vi "Alarme_Geral.vi"() -> ()   [LabVIEW 2019]
panel:
  out "ALARME":bool
  in  "CODIGO":string
  out "DESCRI敲O DO ERRO:":string
  out "STR_ALARME:":string
  in  "[ESC]":bool
  # "ALARME"
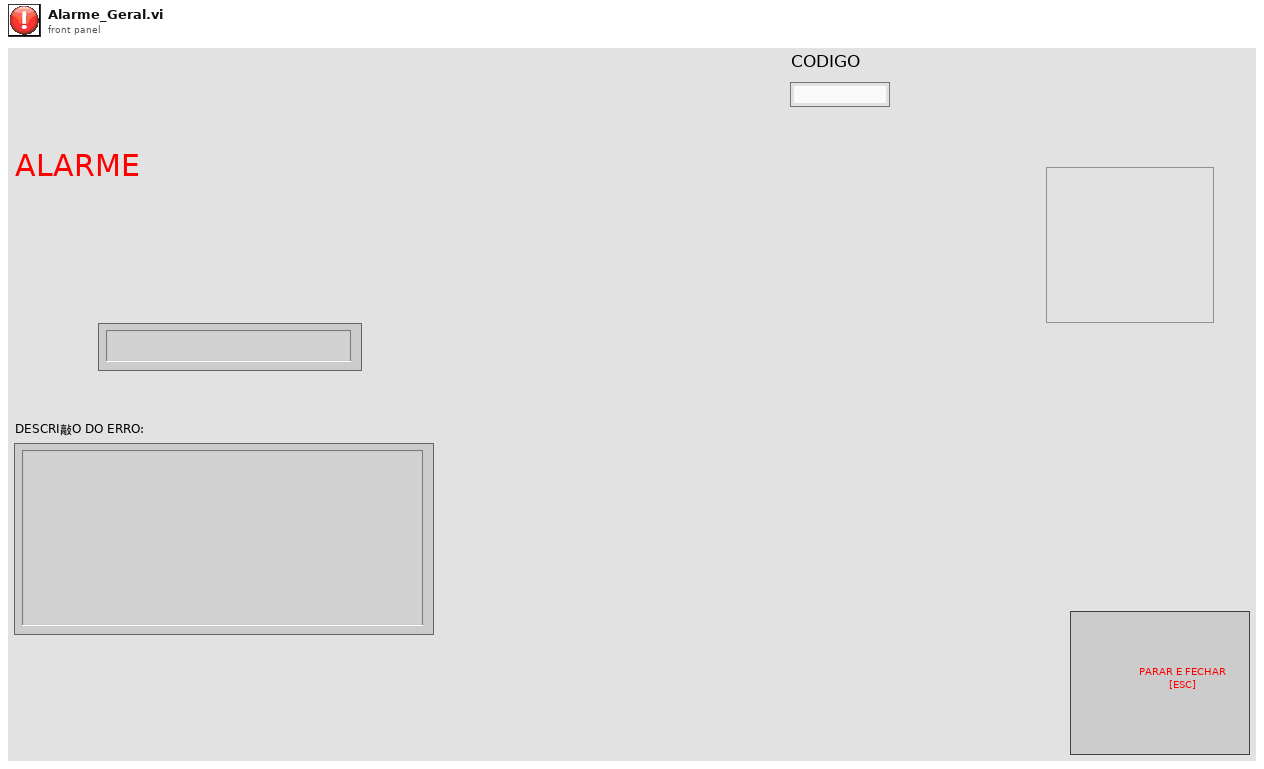
[diagram p1: front panel]
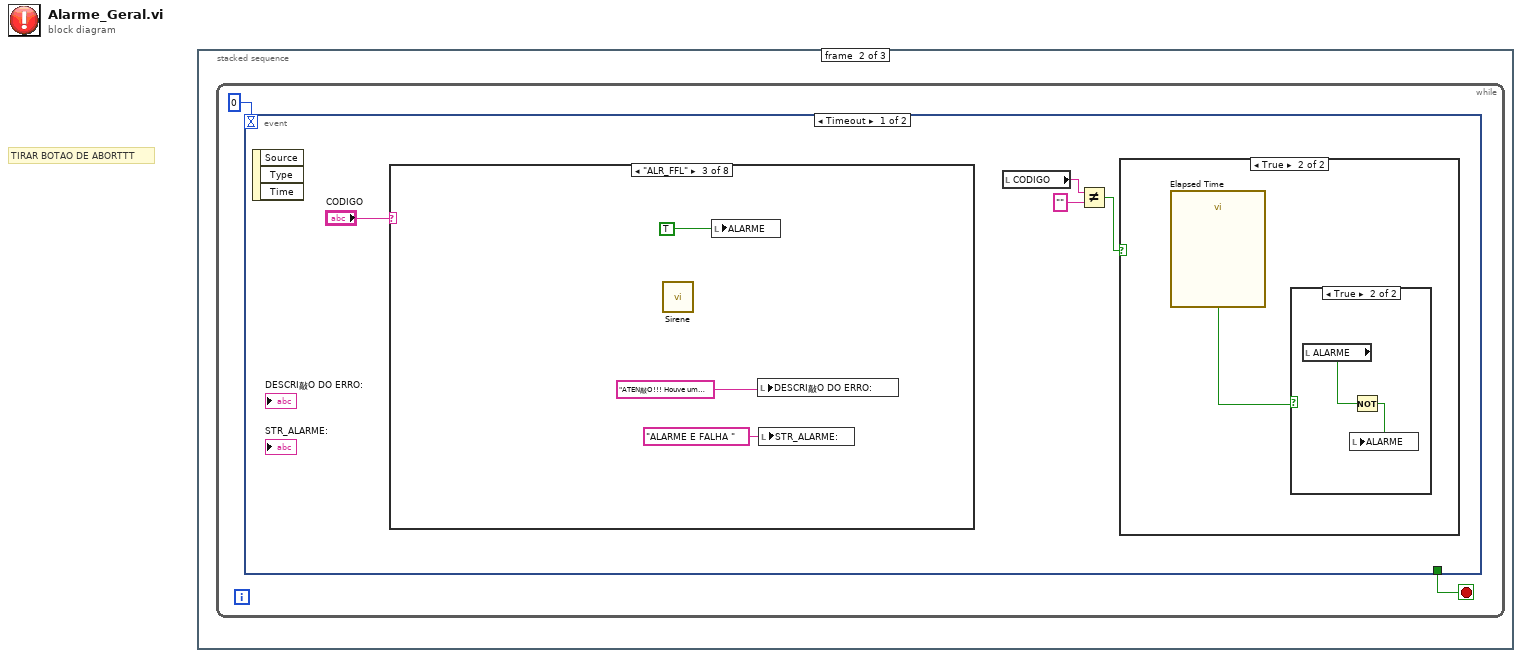
[diagram p0: block diagram]
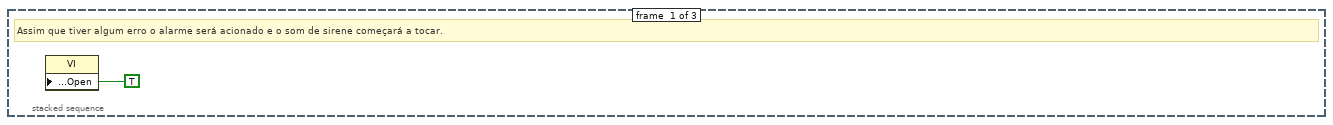
[diagram p2: hidden frame]
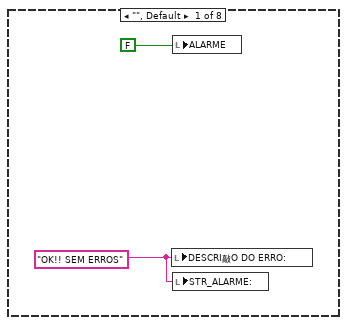
[diagram p5: hidden frame]
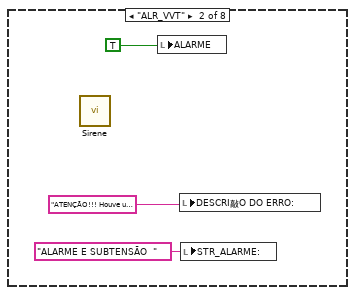
[diagram p6: hidden frame]
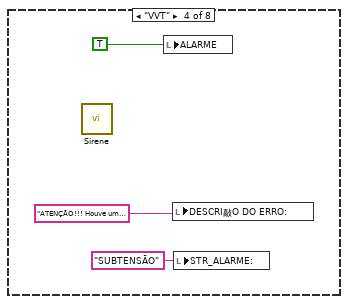
[diagram p7: hidden frame]
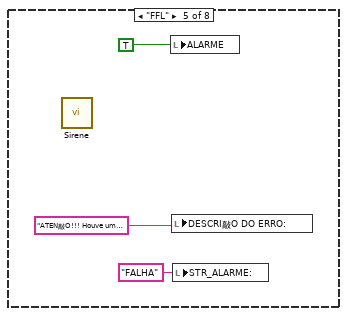
[diagram p8: hidden frame]
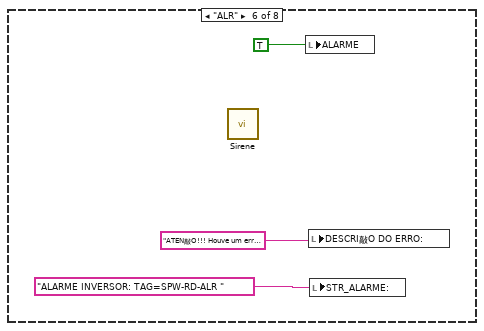
[diagram p9: hidden frame]
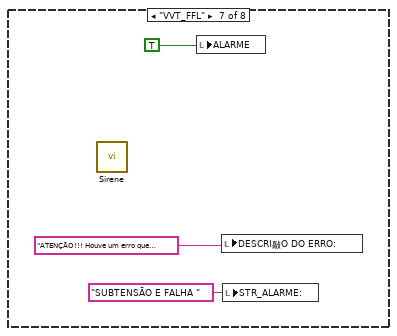
[diagram p10: hidden frame]
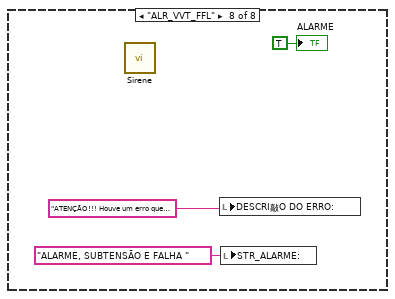
[diagram p11: hidden frame]
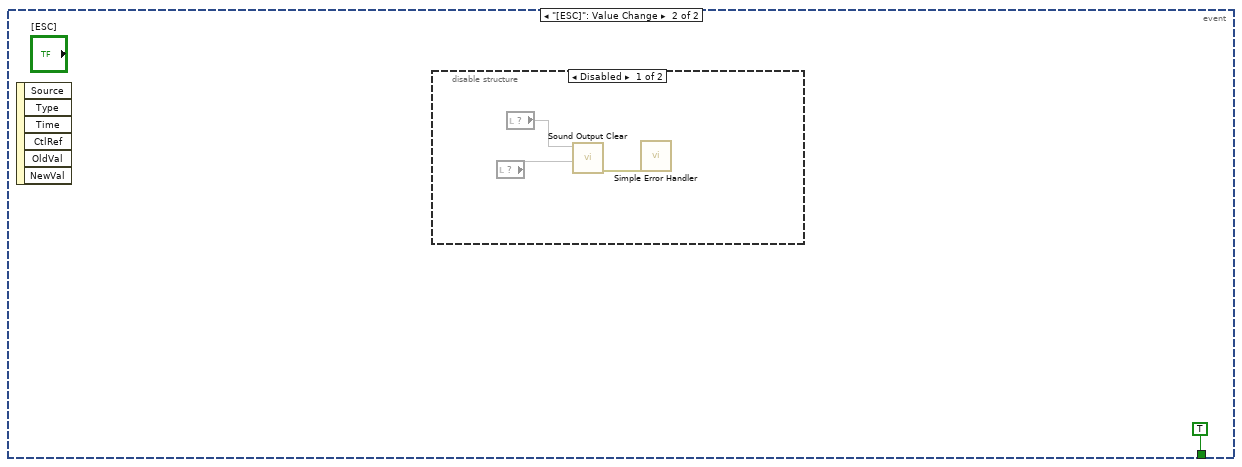
[diagram p12: hidden frame]
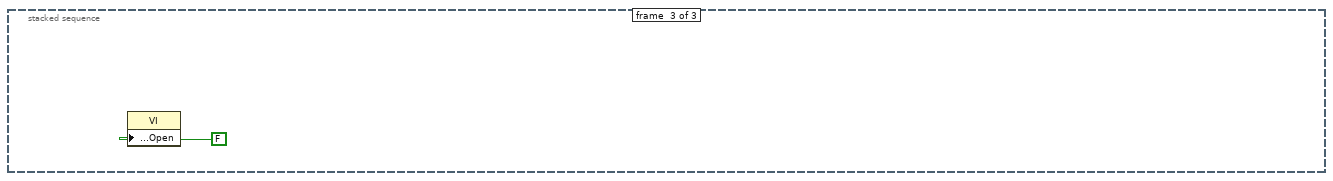
[diagram p14: hidden frame]
diagram:
  # "TIRAR BOTAO DE ABORTTT"
  n1 = stacked-sequence {
    frame #0 {
      # "Assim que tiver algum erro o alarme será acionado e o som de sirene começará a tocar."
      n2 = property class="VI"("Front Panel.Open"=TRUE ("Front Panel Window:Open")) -> ()  [unwired: 2 in, 2 out]
    }
    frame #1 {
      n3 = while {
        stop <- w2 stop-if-true
        n4 = event shown="[0] Timeout" {
          selector: _ -> [_ _]
          dyn-events: _ -> [_ _]
          timeout: 0 -> [_ _]
          tunnel: [_ TRUE] -> w2
          event Timeout {
            n5 = event-data() -> ()  [unwired: 1 in, 3 out]
            n6 = case shown="\"ALR_FFL\"" "CODIGO" {
              frame "", Default {
                w11 = "OK!! SEM ERROS" ("DESCRI敲O DO ERRO:")
                n7 = local write "DESCRI敲O DO ERRO:"(w11) -> ()
                n8 = local write "ALARME"(FALSE ("Alarme_button")) -> ()
                n9 = local write "STR_ALARME:"(w11) -> ()
              }
              frame "ALR_VVT" {
                n10 = call "Sirene.vi"() -> ()  [unwired: 12 in]
                n11 = local write "ALARME"(TRUE ("Alarme_button")) -> ()
                n12 = local write "DESCRI敲O DO ERRO:"("ATENÇÃO!!! Houve um erro que disparou o alarme e o alerta de subtensão. Cheque os parametros e as possiveis causas. " ("DESCRI敲O DO ERRO:")) -> ()
                n13 = local write "STR_ALARME:"("ALARME E SUBTENSÃO  " ("STR_ALARME:")) -> ()
              }
              frame "ALR_FFL" {
                n14 = call "Sirene.vi"() -> ()  [unwired: 12 in]
                n15 = local write "ALARME"(TRUE ("Alarme_button")) -> ()
                n16 = local write "DESCRI敲O DO ERRO:"("ATEN敲O!!! Houve um erro que disparou o alarme e a falha. Cheque os parametros e as possiveis causas. " ("DESCRI敲O DO ERRO:")) -> ()
                n17 = local write "STR_ALARME:"("ALARME E FALHA " ("STR_ALARME:")) -> ()
              }
              frame "VVT" {
                n18 = call "Sirene.vi"() -> ()  [unwired: 12 in]
                n19 = local write "ALARME"(TRUE ("Subtensao_button")) -> ()
                n20 = local write "DESCRI敲O DO ERRO:"("ATENÇÃO!!! Houve um erro que disparou o alerta de subtensão. Cheque os parametros e as possiveis causas. " ("DESCRI敲O DO ERRO:")) -> ()
                n21 = local write "STR_ALARME:"("SUBTENSÃO" ("STR_ALARME:")) -> ()
              }
              frame "FFL" {
                n22 = call "Sirene.vi"() -> ()  [unwired: 12 in]
                n23 = local write "ALARME"(TRUE ("Alarme_button")) -> ()
                n24 = local write "DESCRI敲O DO ERRO:"("ATEN敲O!!! Houve um erro que disparou a falha. Cheque os parametros e as possiveis causas. " ("DESCRI敲O DO ERRO:")) -> ()
                n25 = local write "STR_ALARME:"("FALHA" ("STR_ALARME:")) -> ()
              }
              frame "ALR" {
                n26 = call "Sirene.vi"() -> ()  [unwired: 12 in]
                n27 = local write "ALARME"(TRUE ("Alarme_button")) -> ()
                n28 = local write "DESCRI敲O DO ERRO:"("ATEN敲O!!! Houve um erro que disparou o alerta. Cheque os parametros e as possiveis causas. " ("DESCRI敲O DO ERRO:")) -> ()
                n29 = local write "STR_ALARME:"("ALARME INVERSOR: TAG=SPW-RD-ALR " ("STR_ALARME:")) -> ()
              }
              frame "VVT_FFL" {
                n30 = call "Sirene.vi"() -> ()  [unwired: 12 in]
                n31 = local write "ALARME"(TRUE ("Alarme_button")) -> ()
                n32 = local write "DESCRI敲O DO ERRO:"("ATENÇÃO!!! Houve um erro que disparou o alerta de subtensão e falha. Cheque os parametros e as possiveis causas. " ("DESCRI敲O DO ERRO:")) -> ()
                n33 = local write "STR_ALARME:"("SUBTENSÃO E FALHA " ("STR_ALARME:")) -> ()
              }
              frame "ALR_VVT_FFL" {
                n34 = call "Sirene.vi"() -> ()  [unwired: 12 in]
                n35 = local write "DESCRI敲O DO ERRO:"("ATENÇÃO!!! Houve um erro que disparou o alarme, alerta de subtensão e falha. Cheque os parametros e as possiveis causas. " ("DESCRI敲O DO ERRO:")) -> ()
                n36 = local write "STR_ALARME:"("ALARME, SUBTENSÃO E FALHA " ("STR_ALARME:")) -> ()
                "ALARME" <- TRUE ("ALARME")
              }
            }
            n37 = local read "CODIGO"() -> (w6:string)
            n38 = Not Equal?(x=w6, y="") -> (x != y?=w4:bool)
            n39 = case shown="True" w4 {
              frame False {
              }
              frame True {
                n40 = call "Elapsed Time"() -> ("Time has Elapsed"=w8:bool)  [unwired: 12 in, 7 out]
                n41 = case shown="True" w8 {
                  frame False {
                  }
                  frame True {
                    n42 = local read "ALARME"() -> (w10:bool)
                    n43 = Not(x=w10) -> (.not. x?=w9:bool)
                    n44 = local write "ALARME"(w9) -> ()
                  }
                }
              }
            }
          }
          event "[ESC]": Value Change {
            n45 = event-data() -> ()  [unwired: 1 in, 6 out]
            n46 = disable-structure shown="Disabled" {
              frame Disabled {
                n47 = local read item#-1() -> (w35)
                n48 = local read item#-1() -> (w37)
                n49 = call <vilib>:"Sound Output Clear.vi"("error in (no error)"=w35, "task ID"=w37) -> ("error out"=w36:errorcluster)  [unwired: 9 in]
                n50 = call <vilib>:"Simple Error Handler.vi"("error in (no error)"=w36) -> ()  [unwired: 4 in, 5 out]
              }
              frame Enabled {
              }
            }
          }
        }
      }
    }
    frame #2 {
      n51 = property class="VI"("Front Panel.Open"=FALSE ("Front Panel Window:Open")) -> ()  [unwired: 2 in, 2 out]
    }
  }
